vi "TEST-Draft.vi"() -> ()   [LabVIEW 2020, in "CSMStand(Lite)-test.lvlib"]
uses:
  <vilib>/Utility/miscctls.llb/LVBoundsTypeDef.ctl
  <vilib>/Utility/miscctls.llb/LVRowAndColumnTypeDef.ctl
  <vilib>/Utility/miscctls.llb/LVRowAndColumnUnsignedTypeDef.ctl
  CSMStand(Lite)-test.lvlib
panel:
  out "Active Cell:Cell Size":T1
  out "Bounds":T1
  out "Content Rect Bounds":T1
  out "error out":errorcluster
  in  "Multicolumn Listbox":i32(listbox)
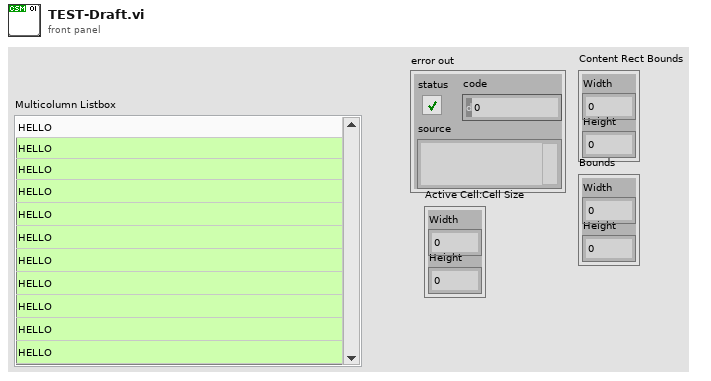
[diagram p1: front panel]
types:
  T1 = typedef "LVBoundsTypeDef.ctl" = cluster{"Width":u32, "Height":u32}
  T2 = typedef "LVRowAndColumnTypeDef.ctl" = cluster{"Row":i32, "Column":i32}
  T3 = typedef "LVRowAndColumnUnsignedTypeDef.ctl" = cluster{"Row":u32, "Column":u32}
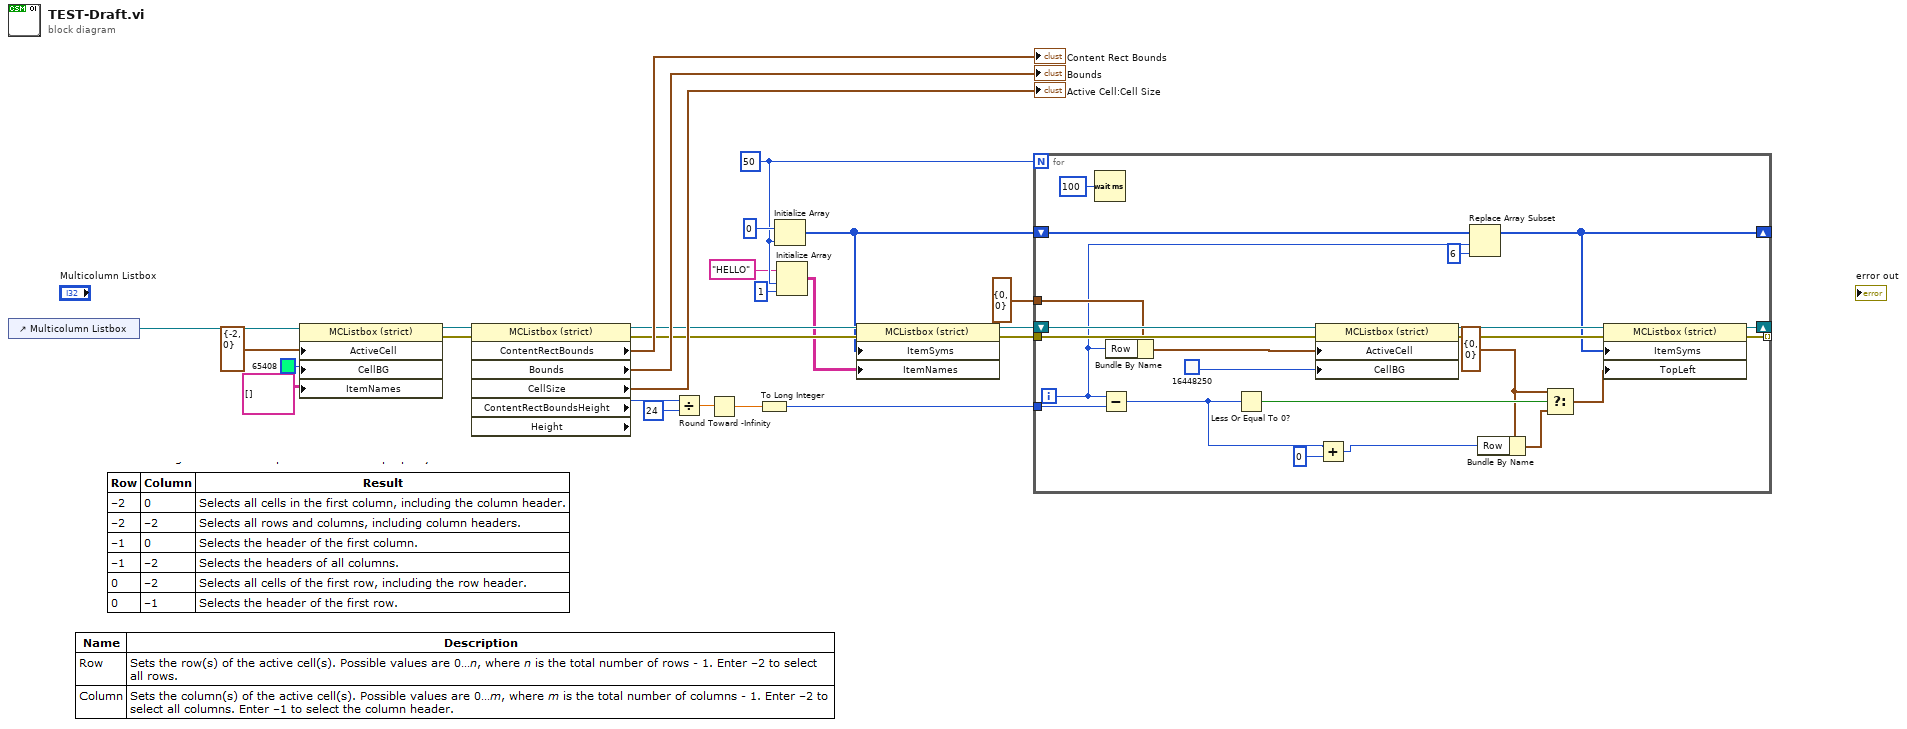
[diagram p0: block diagram]
diagram:
  w5 = 50
  n1 = control-ref of="Multicolumn Listbox"() -> (w23:refnum<vi>)
  n2 = property class="MCListbox (strict)"(reference=w23, "ActiveCell"=T2 {"Row"=-2, "Column"=0} ("Selected Cell"), "CellBG"=u32 65408 ("Selection Color"), "ItemNames"=string[][] [] ("Item Names")) -> (reference out=w22:refnum<vi>, error out=w21:errorcluster)  [unwired: 1 in]
  n3 = property class="MCListbox (strict)" props=["ContentRectBounds", "Bounds", "CellSize", "ContentRectBoundsHeight", "Height"](reference=w22, error in=w21) -> (reference out=w15:refnum<vi>, error out=w7:errorcluster, "ContentRectBounds"=→"Content Rect Bounds":T1, "Bounds"=→"Bounds":T1, "CellSize"=→"Active Cell:Cell Size":T1, "ContentRectBoundsHeight"=w17:i32)  [unwired: 1 out]
  n4 = Divide(x=w17, y=24) -> (x/y=w16:dbl)
  n5 = Round Toward -Infinity(1:w16) -> (0:w14:dbl)
  n6 = To Long Integer(number=w14) -> (32bit integer=w13:i32)
  n7 = Initialize Array(0, w5) -> (w6:i32[])
  n8 = Initialize Array("HELLO", w5, 1 ("dimension size")) -> (w2:string[][])
  n9 = property class="MCListbox (strict)"(reference=w15, error in=w7, "ItemSyms"=w6, "ItemNames"=w2) -> (reference out=w9:refnum<vi>, error out=w8:errorcluster)
  n10 = for {
    N: w5 -> [_]
    shift-right: [w41] -> _
    shift-left: w9 -> [w47]
    tunnel: w8 -> [w46]
    tunnel: w13 -> [w37]
    tunnel: T2 {"Row"=0, "Column"=0} ("Active Cell:Active Cell") -> [w45]
    tunnel: [w38] -> _ mode=indexing
    shift-right: [w30] -> _
    shift-left: w6 -> [w33]
    i -> [w32]
    w35 = T3 {"Row"=0, "Column"=0} ("Top Left Visible Cell")
    n11 = Wait (ms)(milliseconds to wait=u32 100) -> ()  [unwired: 1 out]
    n12 = Subtract(x=w32, y=w37) -> (x-y=w29:i32)
    n13 = Bundle By Name(cluster=w45, "Row"=w32) -> (w44:T2)
    n14 = Less Or Equal To 0?(x=w29) -> (x <= 0?=w36:bool)
    n15 = property class="MCListbox (strict)"(reference=w47, error in=w46, "ActiveCell"=w44, "CellBG"=u32 16448250 ("Selection Color")) -> (reference out=w40:refnum<vi>, error out=w39:errorcluster)
    n16 = Add(x=w29, y=0) -> (x+y=w28:i32)
    n17 = Replace Array Subset(array=w33, new element=6 ("new element/subarray"), index=w32) -> (w30:i32[])
    n18 = Bundle By Name(cluster=w35, "Row"=w28) -> (w34:T3)
    n19 = Select(t=w35, s=w36, f=w34) -> (s? t:f=w26:T3)
    n20 = property class="MCListbox (strict)"(reference=w40, error in=w39, "ItemSyms"=w30, "TopLeft"=w26) -> (reference out=w41:refnum<vi>, error out=w38:errorcluster)
  }
